vi "AngleControl.vi"(11 "anglerUp":bool) -> ()   [LabVIEW 2015]
uses:
  <vilib>/Rock Robotics/WPI/Solenoid/WPI_SolenoidValue.ctl
  <vilib>/Rock Robotics/WPI/Solenoid/WPI_SolenoidSetEnum.vi
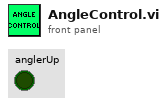
[diagram p1: front panel]
types:
  T1 = typedef "WPI_SolenoidValue.ctl" = enum16{"Off", "On", "Forward", "Reverse"}
  T2 = typedef "WPI_SolenoidDevRef.ctl" = cluster{"DevStatus":errorcluster, "Pneumatics Control Module":u8, "Forward Solenoid Channel":T3, "Reverse Solenoid Channel":T3}
  T3 = typedef "WPI_SolenoidChannel.ctl" = enum8{"Solenoid 0", "Solenoid 1", "Solenoid 2", "Solenoid 3", "Solenoid 4", "Solenoid 5", "Solenoid 6", "Solenoid 7", "Invalid"}
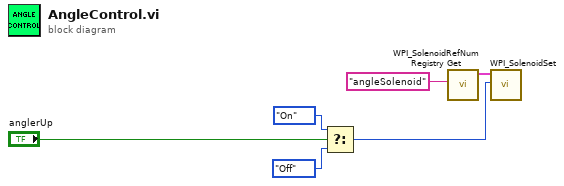
[diagram p0: block diagram]
diagram:
  n1 = Select(t=WPI_SolenoidValue."On" ("Value"), s="anglerUp", f=WPI_SolenoidValue."Off" ("Value")) -> (s? t:f=w1:T1)
  n2 = call <vilib>:"WPI_SolenoidRefNum Registry Get.vi"("refnum name"="angleSolenoid") -> ("SolenoidDevRef"=w4:T2)  [unwired: 9 in, 1 out]
  n3 = call-poly <vilib>:"WPI_SolenoidSet.vi"("Value"=w1, "SolenoidDevRef"=w4) -> ()  [unwired: 8 in, 2 out]
